vi "Update_UI_SelectedOverlayChangeToROI.vi"(8 "error in (no error)":errorcluster, 10 "LstBox Refnum":refnum<vi>, 11 "Image Refnum":refnum<vi>) -> (0 "error out":errorcluster)   [LabVIEW 2019]
uses:
  Controls/ROI_List_Action.ctl
  <vilib>/vision/Image Controls.llb/IMAQ Image.ctl
panel:
  in  "Vision_Image":T1(plugin-control)
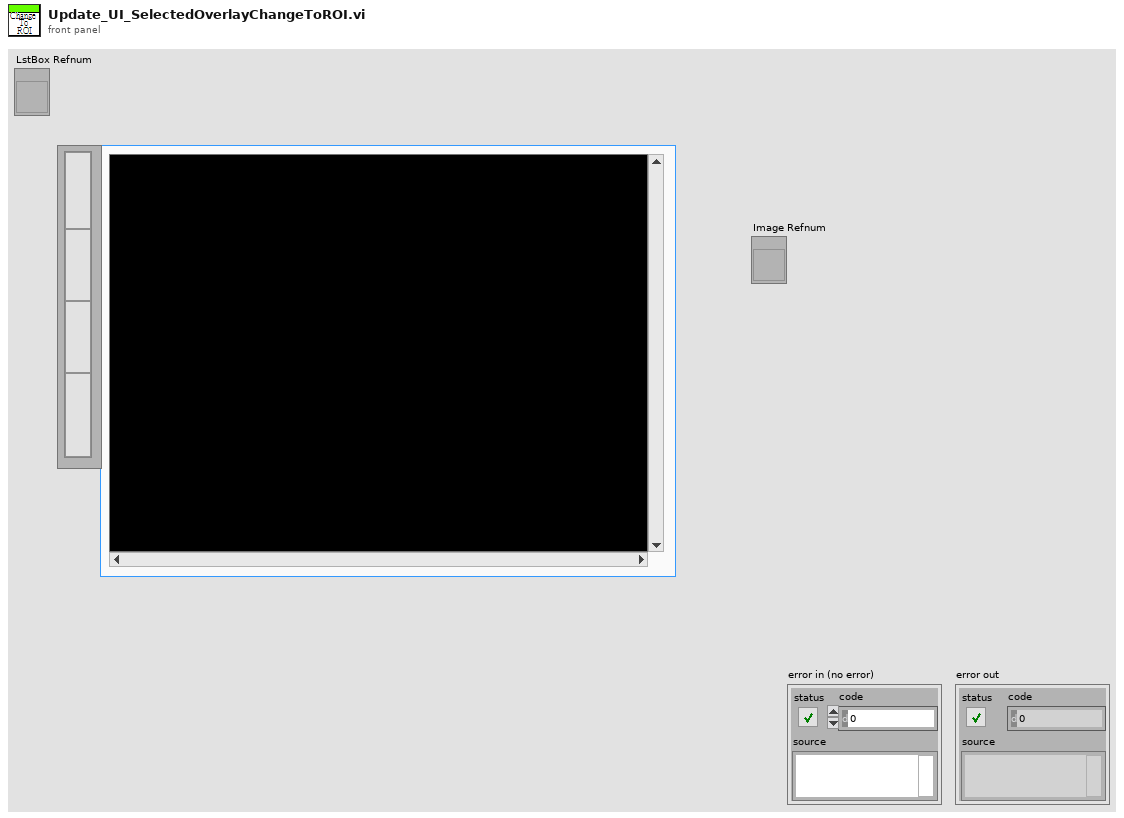
[diagram p1: front panel]
types:
  T1 = typedef "IMAQ Image.ctl" = refnum<image>
  T2 = typedef "ROI_List_Action.ctl" = enum16{"Init", "Add ROI", "Delete ROI", "Get All ROI", "Get Specific ROI", "Set Analysis Setting", "Set Process Setting", "Replace All Entries", "ROIEntryBackup", "ROIEntryBackupClear", "ROIEntryReturn"}
  T3 = cluster{"Contour Type":u32, "ROI Type":i32, "Points":i32[]}
  T4 = cluster{"Global Rectangle":i32[], "Contours":cluster{"Contour Type":u32, "ROI Type":u32, "Points":i32[]}[]}
  T5 = typedef "Vision_DataEntry.ctl" = cluster{"vROIName":string, "vROIContour":cluster{"Contour Type":u32, "ROI Type":u32, "Points":i32[]}, "ProcessSetting":T6[], "Analysis_Setting":T8}
  T6 = typedef "Process_Setting.ctl" = cluster{"Enum_PreProcess":T7, "Parameter":string}
  T7 = typedef "VisionProcessName.ctl" = enum16{"*CamParameter*", "CamAttributes", "*Preprocess*", "CG_Brightness", "C_Plane Extraction", "C_Threshold", "G_Lookup Table", "G_Threshold"}
  T8 = typedef "Analysis_Setting.ctl" = cluster{"PreProcess":T9, "Parameter":string}
  T9 = typedef "V_Analysis_Type.ctl" = enum16{"None", "C_Color Pattern Matching", "G_PatternMatching", "G_ShapeDectect", "G_GeometricMatch", "B_Area Check"}
  T10 = cluster{"Points[0]":i32, "Points[1]":i32, "Points[2]":i32, "Points[3]":i32}
  T11 = cluster{"Contour Type":u32, "ROI Type":i32, "Points":i32[]}[]
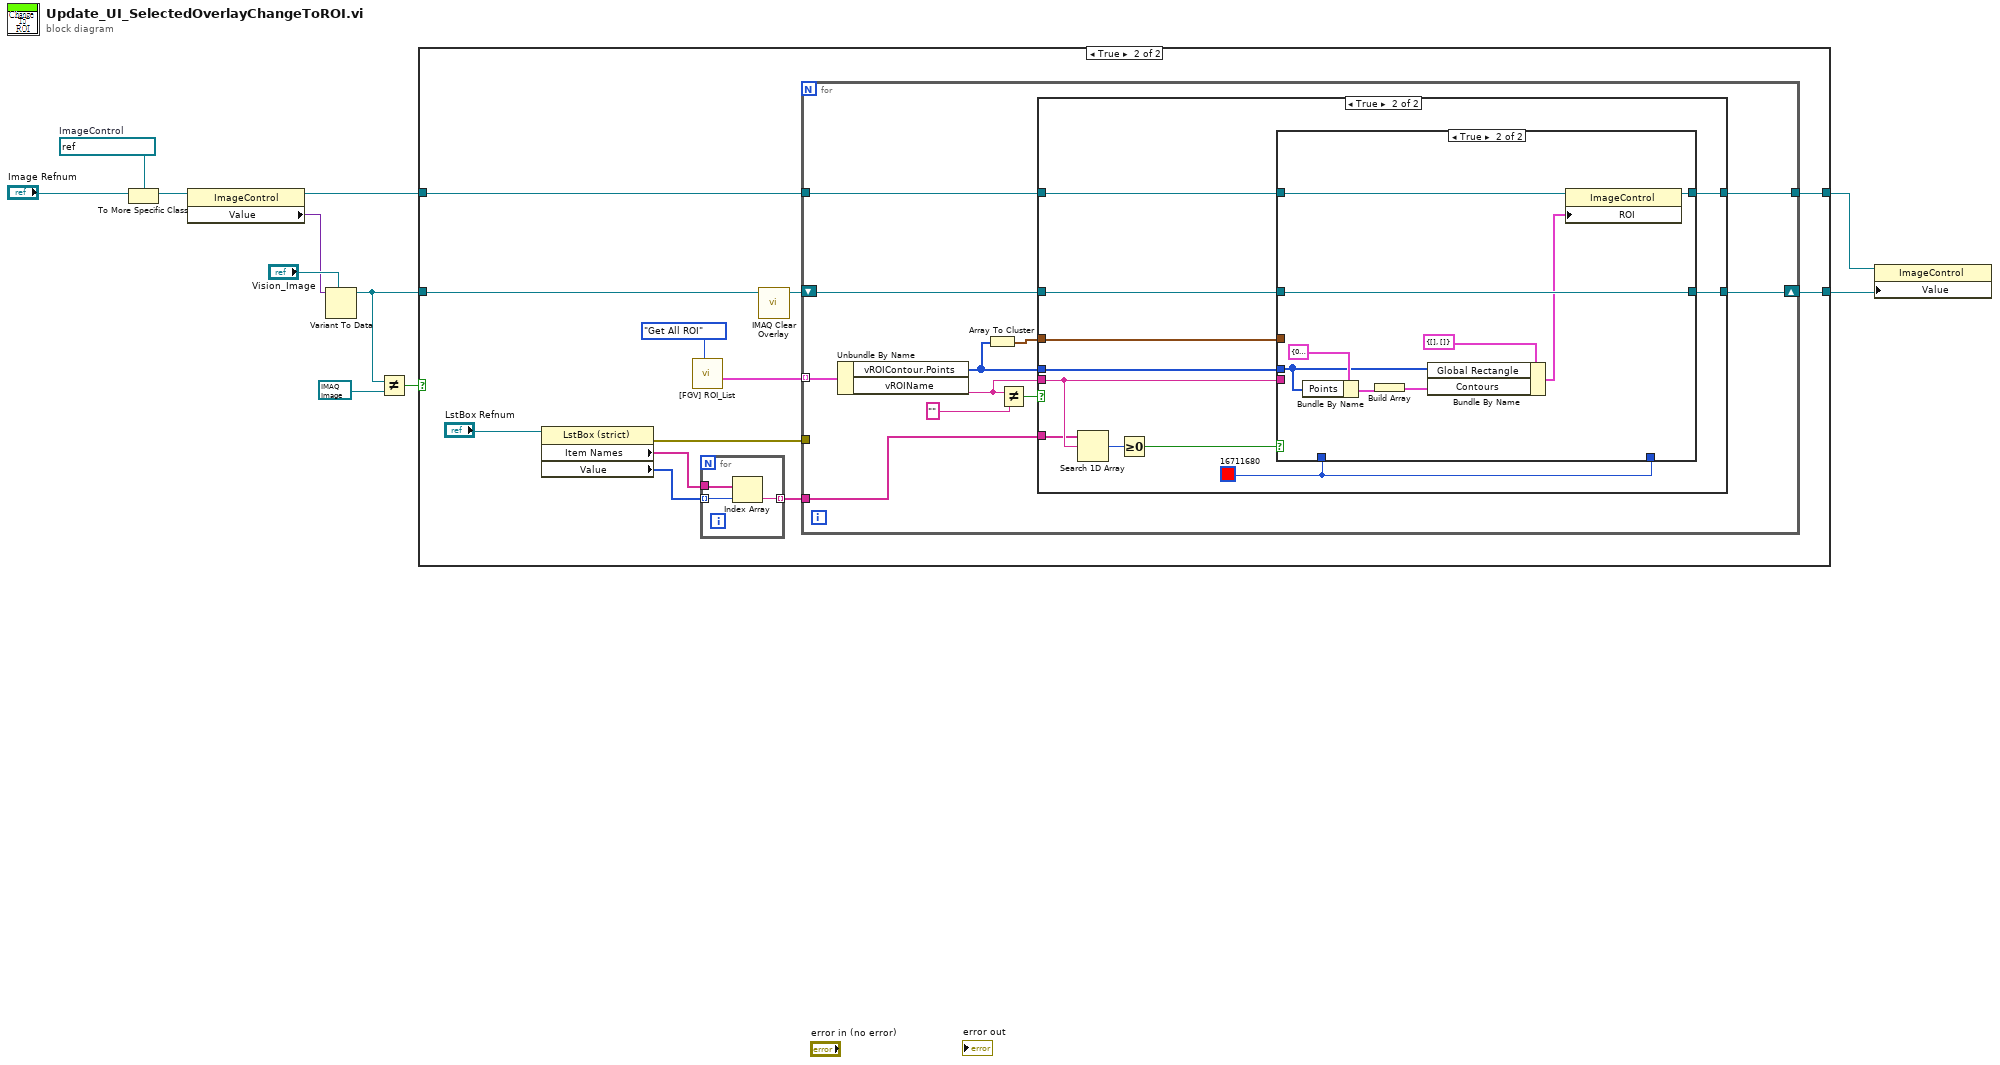
[diagram p0: block diagram]
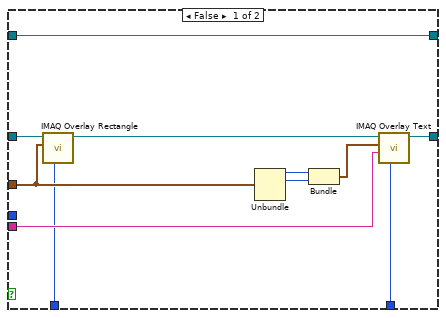
[diagram p4: hidden frame]
diagram:
  w10 = refnum<vi> refnum  # ImageControl
  n1 = To More Specific Class(target class=w10, reference="Image Refnum") -> (specific class reference=w6:refnum<vi>)  [unwired: 1 in, 1 out]
  n2 = property class="ImageControl"(reference=w6) -> (reference out=w2:refnum<vi>, "Value"=w8:variant)  [unwired: 1 in, 1 out]
  n3 = Variant To Data(type="Vision_Image", Variant=w8) -> (data=w3:T1)  [unwired: 1 in, 1 out]
  n4 = Not Equal?(x=w3, y=T1 refnum ("Image Out")) -> (x != y?=w4:bool)
  n5 = case shown="True" w4 {
    tunnel: w3 -> [w13 w24]
    tunnel: [w13 w20] -> w7
    tunnel: w2 -> [w12 w15]
    tunnel: [w12 w14] -> w1
    frame False {
    }
    frame True {
      n6 = property class="LstBox (strict)"(reference="LstBox Refnum") -> (error out=w19:errorcluster, "Item Names"=w17:string[], "Value"=w18:i32[])  [unwired: 1 in, 1 out]
      n7 = call "[FGV] ROI_List.vi"("Action"=ROI_List_Action."Get All ROI") -> ("All ROI"=w21:T5[])  [unwired: 8 in, 2 out]
      n8 = for {
        tunnel: w18 -> [w28] mode=indexing
        tunnel: w17 -> [w27]
        tunnel: [w26] -> w16 mode=indexing
        n9 = Index Array(array=w27, index=w28) -> (element=w26:string)
      }
      n10 = call "IMAQ Clear Overlay"("Image"=w24) -> ("Image Out"=w23:T1)  [unwired: 9 in, 1 out]
      n11 = for {
        tunnel: w21 -> [w37] mode=indexing
        shift-right: [w38] -> w20
        shift-left: w23 -> [w39]
        tunnel: w19 -> [_]
        tunnel: w16 -> [w32]
        tunnel: w15 -> [w31]
        tunnel: [w30] -> w14
        n12 = Unbundle By Name(w37) -> ("vROIContour.Points"=w29:i32[], "vROIName"=w33:string)
        n13 = Array To Cluster(array=w29) -> (cluster=w34:T10)
        n14 = Not Equal?(x=w33, y="") -> (x != y?=w35:bool)
        n15 = case shown="True" w35 {
          tunnel: w39 -> [w41 w43]
          tunnel: [w41 w52] -> w38
          tunnel: w34 -> [_ w51]
          tunnel: w33 -> [_ w50]
          tunnel: w32 -> [_ w49]
          tunnel: w31 -> [w40 w46]
          tunnel: [w40 w45] -> w30
          tunnel: w29 -> [_ w44]
          frame False {
          }
          frame True {
            w42 = u32 16711680 ("Color")
            n16 = Search 1D Array(1D array=w49, element=w50) -> (index of element=w48:i32)  [unwired: 1 in]
            n17 = Greater Or Equal To 0?(x=w48) -> (x >= 0?=w47:bool)
            n18 = case shown="True" w47 {
              tunnel: w43 -> [w56 w70]
              tunnel: [w60 w70] -> w52
              tunnel: w51 -> [w54 _]
              tunnel: w42 -> [w59 _]
              tunnel: w50 -> [w58 _]
              tunnel: w46 -> [w57 w72]
              tunnel: [w57 w71] -> w45
              tunnel: w44 -> [_ w67]
              tunnel: w42 -> [w53 _]
              frame False {
                n19 = call "IMAQ Overlay Rectangle"("Color"=w53, "Rectangle"=w54, "Image"=w56) -> ("Image Out"=w55:T1)  [unwired: 7 in, 1 out]
                n20 = Unbundle(w54) -> ("Points[0]"=w63:i32, "Points[1]"=w62:i32)  [unwired: 2 out]
                n21 = Bundle("Points[0]"=w63, "Points[1]"=w62) -> (w61:cluster{"Points[0]":i32, "Points[1]":i32})  [unwired: 1 in]
                n22 = call "IMAQ Overlay Text"("Text Color (black)"=w59, "String"=w58, "Origin"=w61, "Image"=w55) -> ("Image Out"=w60:T1)  [unwired: 6 in, 1 out]
              }
              frame True {
                n23 = Bundle By Name(cluster=T3 {"Contour Type"=0, "ROI Type"=3, "Points"=[]}, "Points"=w67) -> (w66:T3)
                n24 = Build Array(w66) -> (w65:T11)
                n25 = Bundle By Name(cluster=T4 {"Global Rectangle"=[], "Contours"=[]} ("ROI"), "Global Rectangle"=w67, "Contours"=w65) -> (w64:T4)
                n26 = property class="ImageControl"(reference=w72, "ROI"=w64) -> (reference out=w71:refnum<vi>)  [unwired: 1 in, 1 out]
              }
            }
          }
        }
      }
    }
  }
  n27 = property class="ImageControl"(reference=w1, "Value"=w7) -> ()  [unwired: 1 in, 2 out]
